vi "评分系统.vi"() -> ()   [LabVIEW 2018]
panel:
  out "通过或未通过":dbl
  out "指示灯":bool
  in  "x":i32
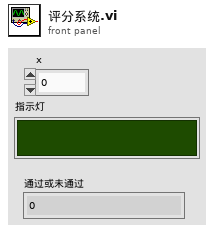
[diagram p1: front panel]
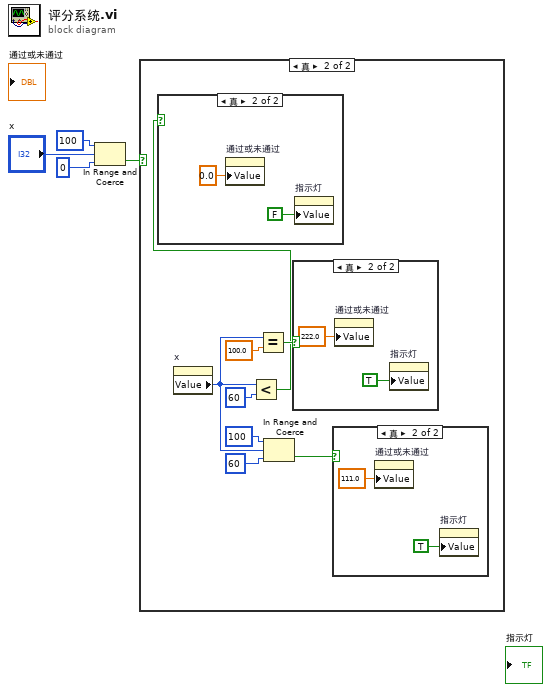
[diagram p0: block diagram]
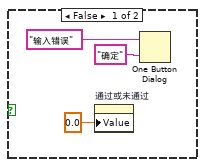
[diagram p2: hidden frame]
diagram:
  n1 = In Range and Coerce(upper limit=100 ("上限"), x="x", lower limit=0 ("下限")) -> (In Range?=w1:bool)  [unwired: 1 out]
  n2 = case shown="真" w1 {
    frame False {
      n3 = property on="通过或未通过" class="DigNum (严格)"("Value"=0.0 ("通过或未通过")) -> ()  [unwired: 2 in, 2 out]
      n4 = One Button Dialog(message="输入错误" ("消息"), button name ("OK")="确定" ("按钮名称（“确定”）")) -> ()  [unwired: 1 out]
    }
    frame True {
      n5 = property on="x" class="DigNum (严格)"() -> ("Value"=w10:i32)  [unwired: 2 in, 2 out]
      n6 = Less?(x=w10, y=60) -> (x < y?=w8:bool)
      n7 = case shown="真" w8 {
        frame False {
        }
        frame True {
          n8 = property on="通过或未通过" class="DigNum (严格)"("Value"=0.0 ("通过或未通过")) -> ()  [unwired: 2 in, 2 out]
          n9 = property on="指示灯" class="Bool (严格)"("Value"=FALSE ("指示灯")) -> ()  [unwired: 2 in, 2 out]
        }
      }
      n10 = Equal?(x=w10, y=100.0) -> (x = y?=w9:bool)
      n11 = In Range and Coerce(upper limit=100 ("上限"), x=w10, lower limit=60 ("下限")) -> (In Range?=w12:bool)  [unwired: 1 out]
      n12 = case shown="真" w9 {
        frame False {
        }
        frame True {
          n13 = property on="通过或未通过" class="DigNum (严格)"("Value"=222.0 ("通过或未通过")) -> ()  [unwired: 2 in, 2 out]
          n14 = property on="指示灯" class="Bool (严格)"("Value"=TRUE ("指示灯")) -> ()  [unwired: 2 in, 2 out]
        }
      }
      n15 = case shown="真" w12 {
        frame False {
        }
        frame True {
          n16 = property on="通过或未通过" class="DigNum (严格)"("Value"=111.0 ("通过或未通过")) -> ()  [unwired: 2 in, 2 out]
          n17 = property on="指示灯" class="Bool (严格)"("Value"=TRUE ("指示灯")) -> ()  [unwired: 2 in, 2 out]
        }
      }
    }
  }
